vi "Keithley 6514 Read Event Register.vi"(0 "Resource In":refnum<visa-resource-name>, 1 "Check For SCPI Errors? (T)":bool=TRUE, 7 "Event Register to Read (Measurement:0)":u16(ring) items=["Measurement", "Operation", "Questionable"], 11 "error in (no error)":T1) -> (4 "Resource Out (dupl)":refnum<visa-resource-name>, 8 "Register Value":u32 max=65535 step=1 format="%016b", 15 "error out":T1)   [LabVIEW 2014, in "KE6514Driver.lvlib"]
doc: "This VI is used to enable the various registers of the 6514.\n\nRegister to Read:\n0 = Measurement\n1 = Operation\n2 = Questionable\n\nRefer to the Users Manual for complete description of the registers and associated bit values."
uses:
  KE6514Driver.lvlib
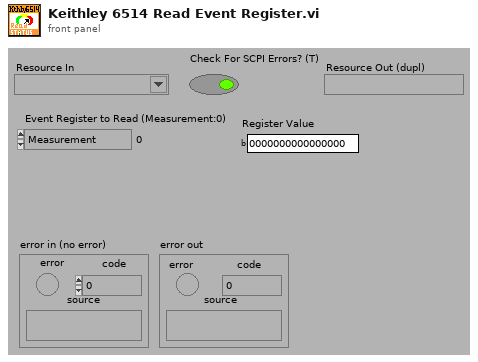
[diagram p1: front panel]
types:
  T1 = cluster{"error":bool, "code":i32, "source":string}
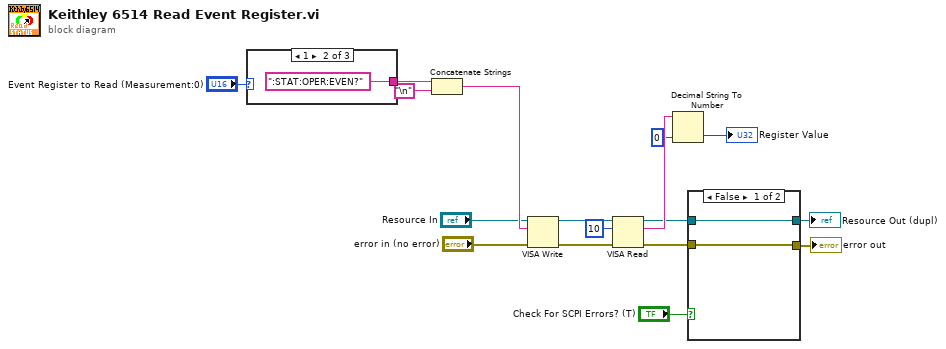
[diagram p0: block diagram]
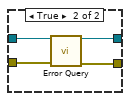
[diagram p2: hidden frame]
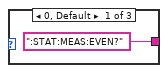
[diagram p3: hidden frame]
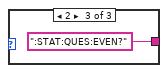
[diagram p4: hidden frame]
diagram:
  n1 = case shown="1" "Event Register to Read (Measurement:0)" {
    tunnel: [":STAT:MEAS:EVEN?" ":STAT:OPER:EVEN?" ":STAT:QUES:EVEN?"] -> w15
    frame 0, Default {
    }
    frame 1 {
    }
    frame 2 {
    }
  }
  n2 = Concatenate Strings(w15, "\n") -> (w13:string)
  n3 = VISA Write(VISA resource name="Resource In", write buffer=w13, error in (no error)="error in (no error)") -> (VISA resource name out=w9:refnum<visa-resource-name>, error out=w10:errorcluster)  [unwired: 1 out]
  n4 = VISA Read(VISA resource name=w9, byte count=u32 10, error in (no error)=w10) -> (VISA resource name out=w4:refnum<visa-resource-name>, read buffer=w7:string, error out=w3:errorcluster)  [unwired: 1 out]
  n5 = Decimal String To Number(string=w7, default (0L)=u32 0 ("default (0 I32)")) -> (number=→"Register Value":u32)  [unwired: 1 in, 1 out]
  n6 = case shown="False" "Check For SCPI Errors? (T)" {
    tunnel: w4 -> [w22 w26]
    tunnel: w3 -> [w21 w25]
    tunnel: [w22 w24] -> w2
    tunnel: [w21 w23] -> w1
    frame False {
    }
    frame True {
      n7 = call "Error Query.vi"("VISA Resource In"=w26, "error in (no error)"=w25) -> ("VISA Resource Out (dupl)"=w24:refnum<visa-resource-name>, "error out"=w23:errorcluster)  [unwired: 10 in, 2 out]
    }
  }
  "error out" <- w1
  "Resource Out (dupl)" <- w2
